vi "img.Subtract.vi"(2 "image2 in":u16[][](array[numeric]), 3 "image1 in":u16[][](array[numeric])) -> (0 "Array":u16[][](array[numeric]), 1 "x > y?":bool)   [LabVIEW 2020]
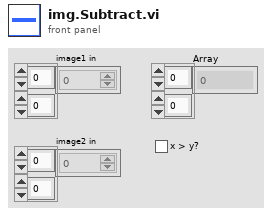
[diagram p1: front panel]
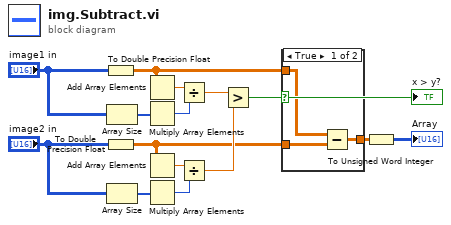
[diagram p0: block diagram]
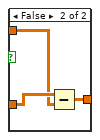
[diagram p2: hidden frame]
diagram:
  n1 = To Double Precision Float(number="image1 in") -> (double precision float=w2:dbl[][])
  n2 = To Double Precision Float(number="image2 in") -> (double precision float=w1:dbl[][])
  n3 = Array Size(array="image1 in") -> (size(s)=w13:i32[])
  n4 = Array Size(array="image2 in") -> (size(s)=w8:i32[])
  n5 = Add Array Elements(numeric array=w2) -> (sum=w11:dbl)
  n6 = Multiply Array Elements(1:w13) -> (0:w12:i32)
  n7 = Add Array Elements(numeric array=w1) -> (sum=w10:dbl)
  n8 = Multiply Array Elements(1:w8) -> (0:w9:i32)
  n9 = Divide(x=w11, y=w12) -> (x/y=w6:dbl)
  n10 = Divide(x=w10, y=w9) -> (x/y=w5:dbl)
  n11 = Greater?(x=w6, y=w5) -> (0:w4:bool)
  "x > y?" <- w4
  n12 = case shown="True" w4 {
    tunnel: [w18 w21] -> w15
    tunnel: w2 -> [w16 w19]
    tunnel: w1 -> [w17 w20]
    frame True {
      n13 = Subtract(x=w16, y=w17) -> (x-y=w18:dbl[][])
    }
    frame False {
      n14 = Subtract(x=w20, y=w19) -> (x-y=w21:dbl[][])
    }
  }
  n15 = To Unsigned Word Integer(number=w15) -> (unsigned 16bit integer=→"Array":u16[][])
